vi "Repeatability_test.vi"(10 "PEU":refnum<class "PEU.lvclass">, 11 "E5071C":refnum<class "E5071C.lvclass">) -> ()   [LabVIEW 2020]
uses:
  Driver/E5071C/E5071C/E5071C.lvclass
  Driver/PEU/PEU/PEU.lvclass
  <vilib>/Math Plots/3D Math Plots/3D Scatter/3D Scatter XCtrl/3D Scatter.xctl
  <vilib>/Utility/NIReport.llb/Report Type.ctl
  Driver/E5071C/E5071C/E5071C.lvclass/E5071C.ctl
  <vilib>/addons/_office/excel.llb/Excel Get Data ([str]).vi
  <vilib>/Math Plots/3D Math Plots/3D Scatter/3D Scatter Datatype/Public/Plot Helper (Matrix).vi
  <vilib>/Utility/NIReport.llb/NI_report.lvclass
  <vilib>/Utility/NIReport.llb/NI_ReportGenerationCore.lvlib
  <vilib>/Utility/NIReport.llb/Excel/NI_Excel.lvclass
  <vilib>/addons/_office/NI_ReportGenerationToolkit.lvlib
  <instrlib>/Agilent ENA Series/Agilent ENA Series.lvlib
  <vilib>/Math Plots/3D Math Plots/3D Scatter/3D Scatter Datatype/3D Scatter Datatype.lvclass
panel:
  in  "循环次数":i32=1 min=1
  in  "引脚":string(combo)="SPDT"
  in  "Load":bool
  in  "Test":bool
  in  "Save":bool
  in  "负载选择":enum32{"Item 0", "Item 1"}(radio)
  in  "DUT ID:":string
  in  "DUT\n开关类型":string(combo)="SPDT"
  in  "Panel Show":bool
  in  "Tab Control":T1(tab)
  out "VSWR Graph":cluster{"频率":dbl[], dbl[]}[](graph)
  out "IL Graph":cluster{"Freqs":dbl[], "temp_value":dbl[]}[](graph)
  out "ISL Graph":cluster{"Freqs":dbl[], "temp_value":dbl[]}[](graph)
  out "VSWR(3D)":refnum<class "3D Plot Datatype.lvclass">[](xcontrol)
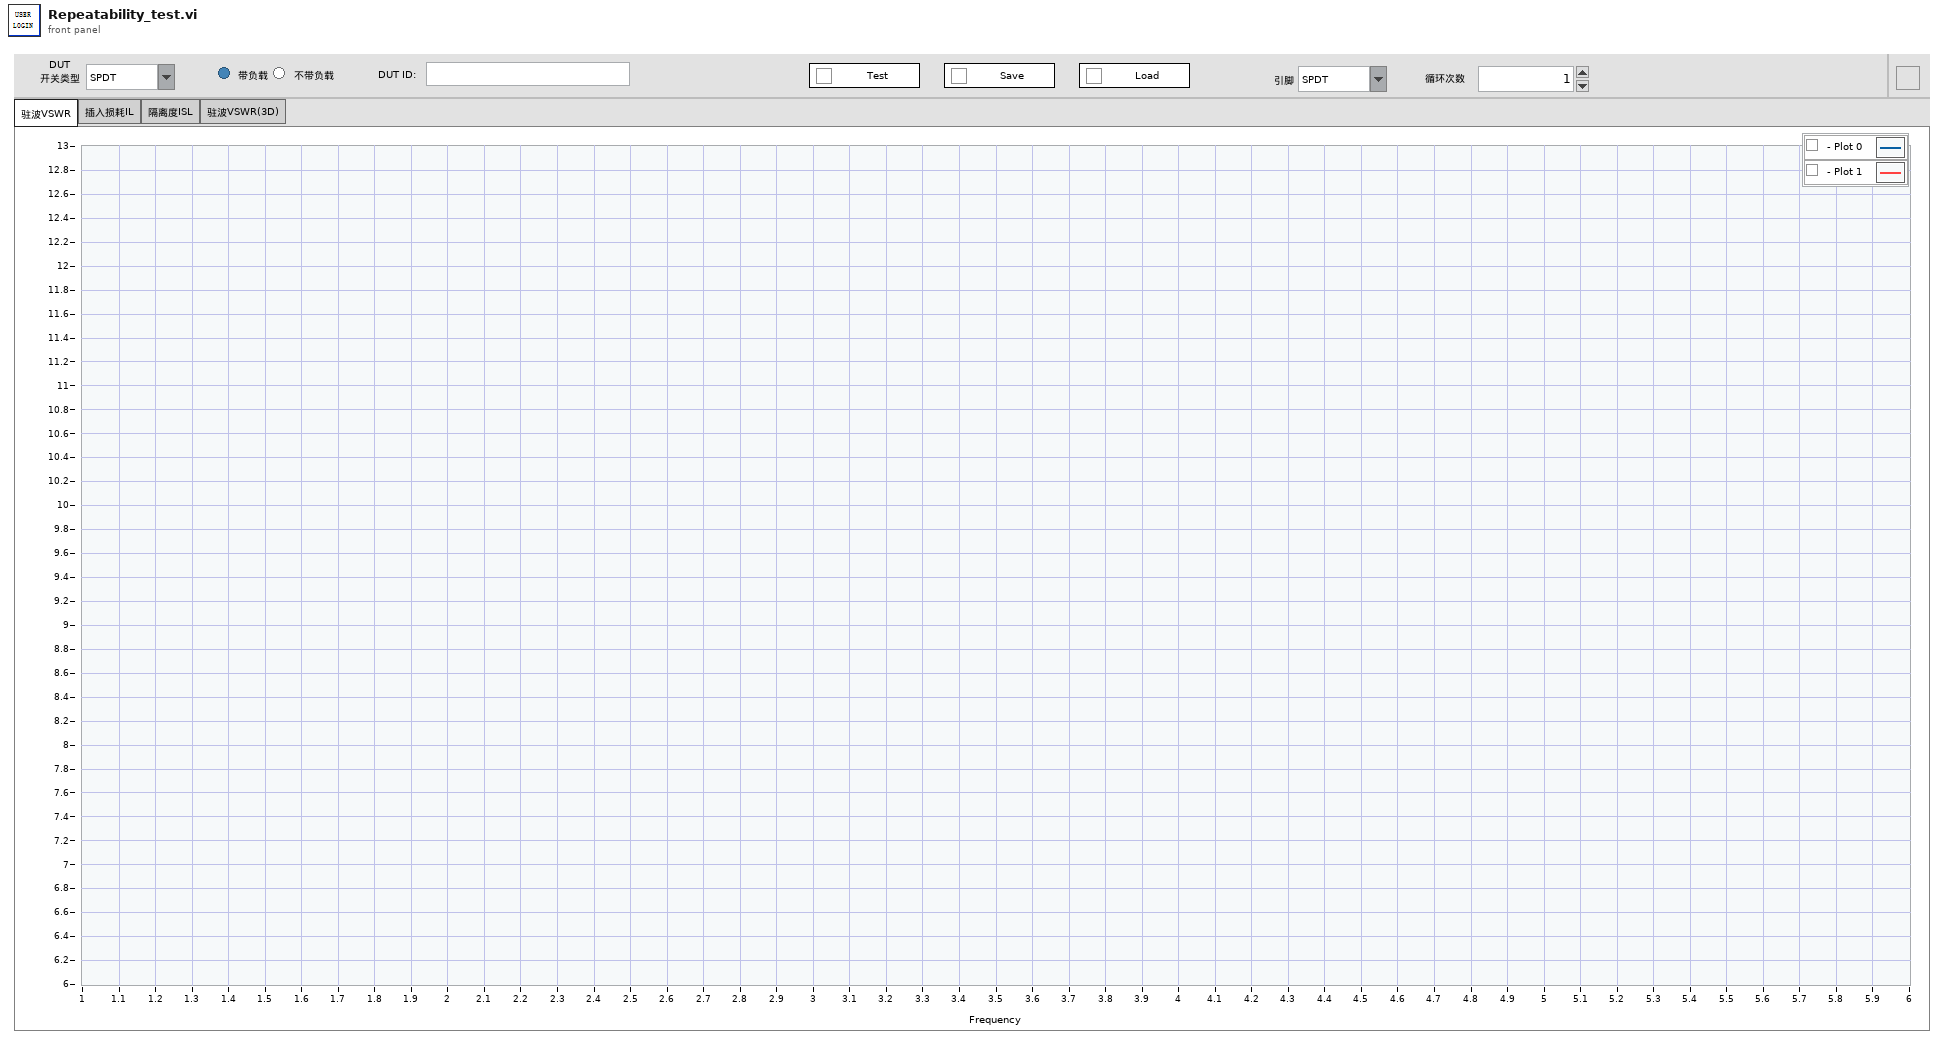
[diagram p1: front panel]
types:
  T1 = enum32{"驻波VSWR", "插入损耗IL", "隔离度ISL", "驻波VSWR(3D)"}
  T2 = enum32{"Invalid", "Standard", "Closed", "Hidden", "Minimized", "Maximized"}
  T3 = cluster{"校准文件":string[], "控制箱通道":string[], "DUT导通引脚":string[], "S名称":string[], "配置S":string[], "Plot_Name":string[]}
  T4 = typedef "NI_ReportGenerationCore.lvlib/Report Type.ctl" = enum16{"HTML", "Word", "Excel"}
  T5 = enum16{"maximized", "minimized", "normal", "no change"}
  T6 = cluster{"E5071C":refnum<class "E5071C.lvclass">, "PEU":refnum<class "PEU.lvclass">, "Index":i32, "Limit_Table":cluster{"Limit_IL":string[][], "Limit_VSWR":string[][], "Limit_ISL":string[][]}, "VSWR Graph":cluster{"频率":dbl[], dbl[]}[], "temp_value":dbl[], "Freqs":dbl[], "Count":i32, "测试逻辑":cluster{"校准文件":string[], "控制箱通道":string[], "DUT导通引脚":string[], "S名称":string[], "配置S":string[], "Plot_Name":string[]}, "VSWR_State":bool, "IL_State":bool, "ISL_State":bool, "循环次数":i32}
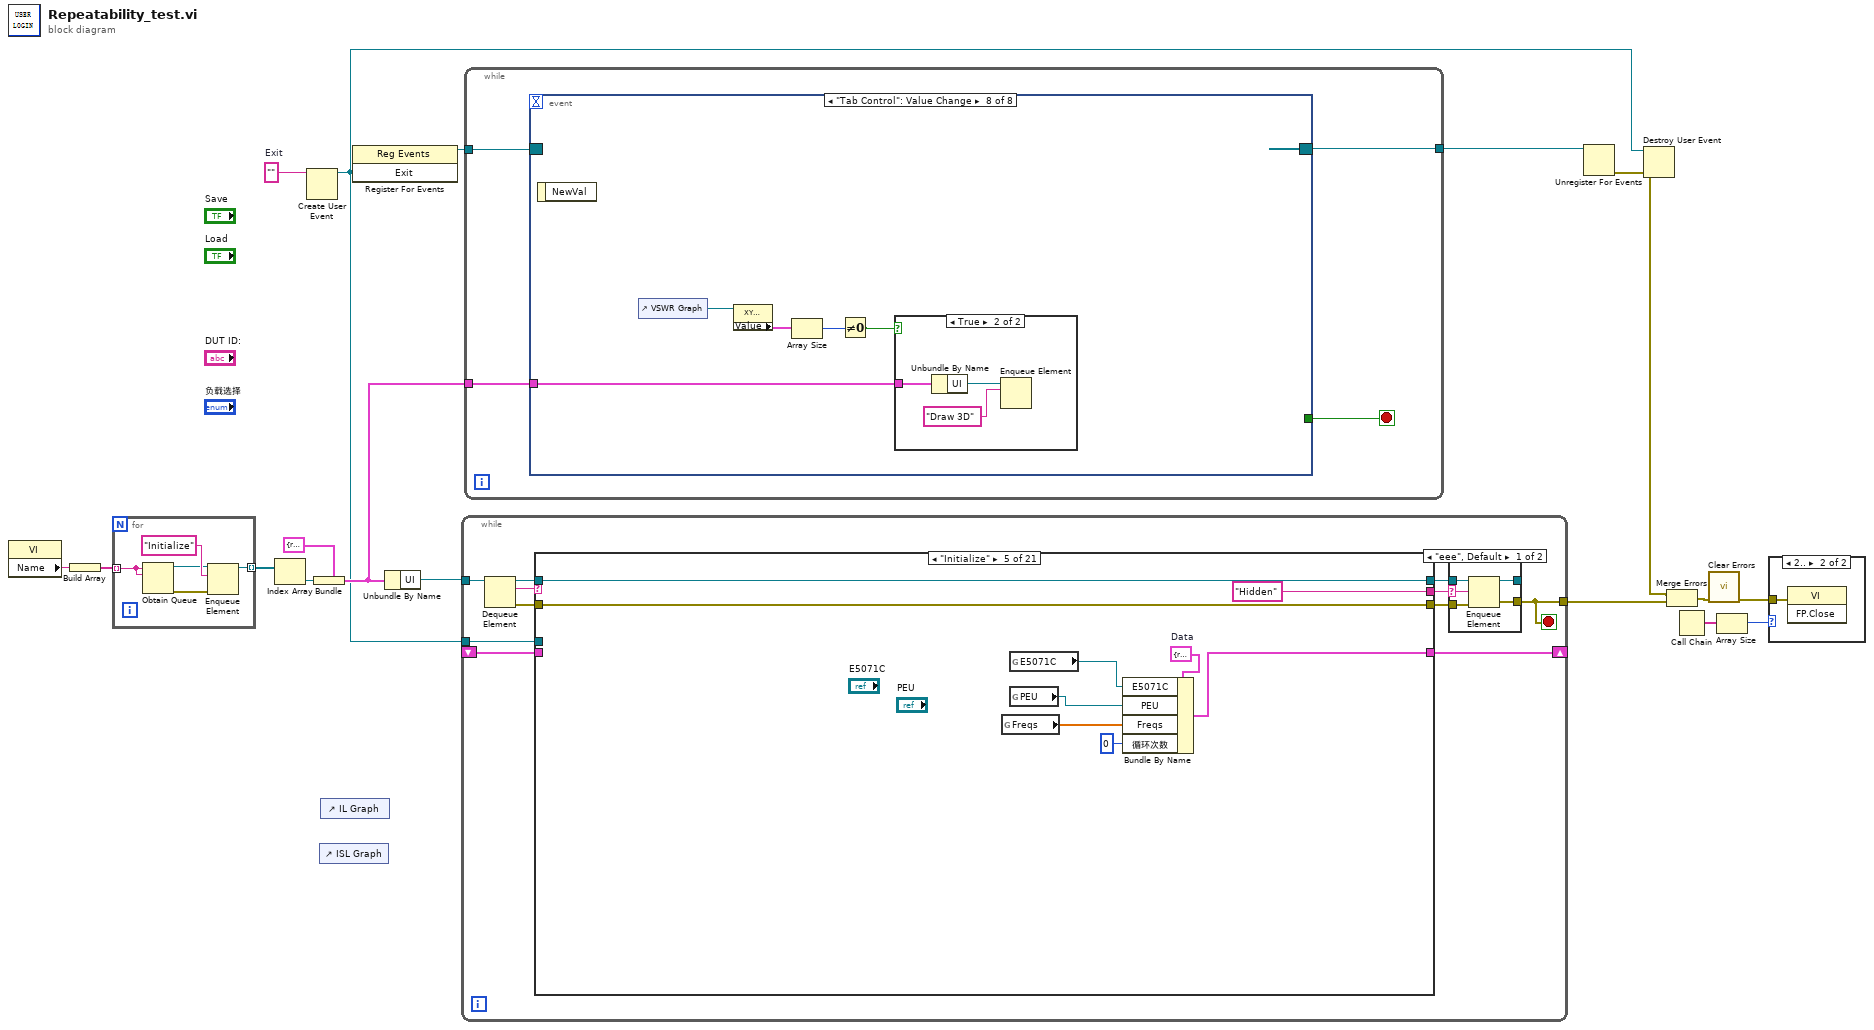
[diagram p0: block diagram]
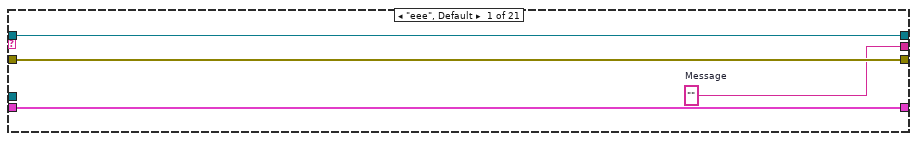
[diagram p4: hidden frame]
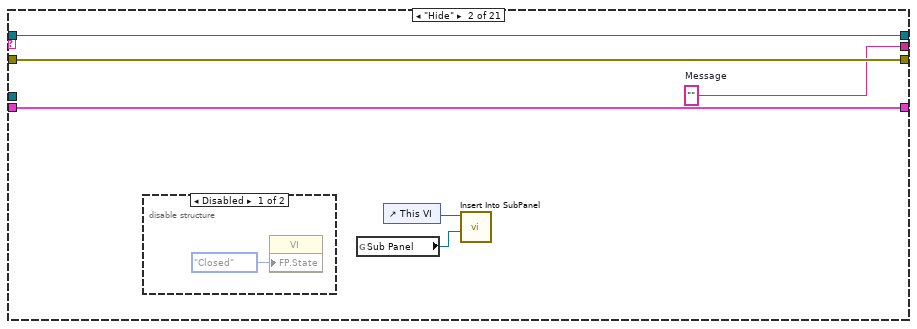
[diagram p5: hidden frame]
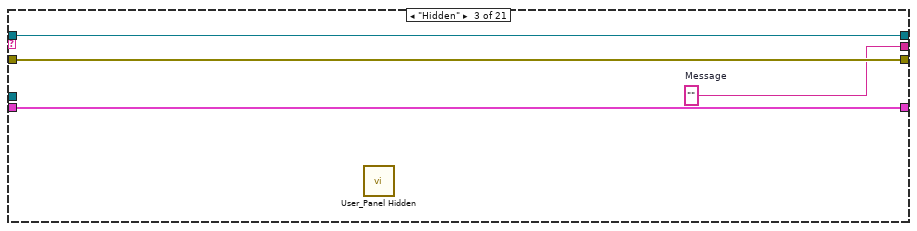
[diagram p7: hidden frame]
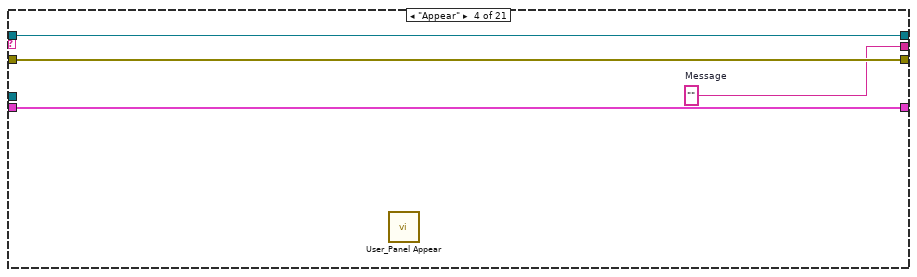
[diagram p8: hidden frame]
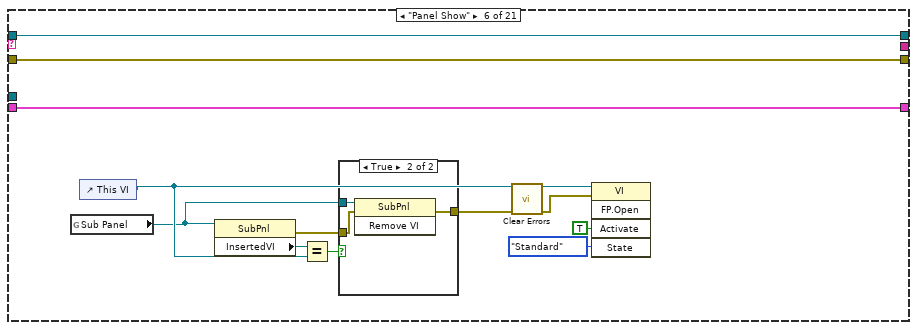
[diagram p9: hidden frame]
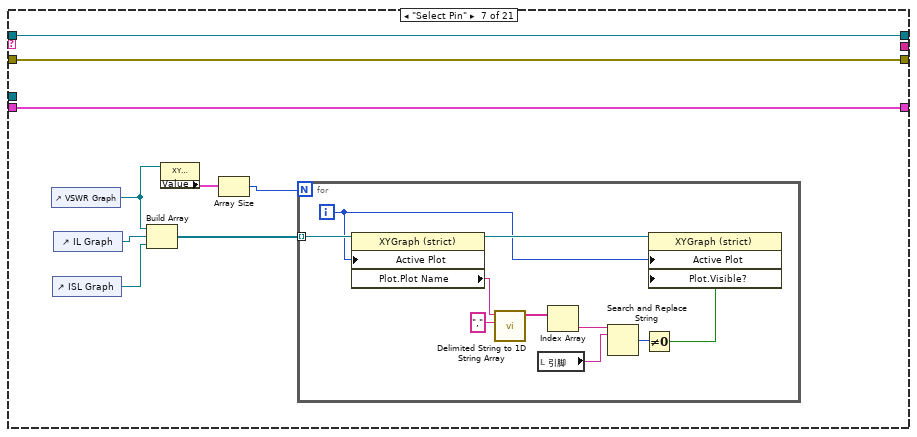
[diagram p11: hidden frame]
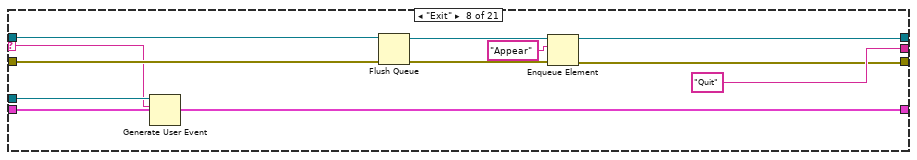
[diagram p12: hidden frame]
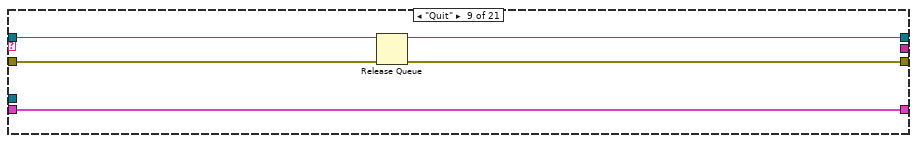
[diagram p13: hidden frame]
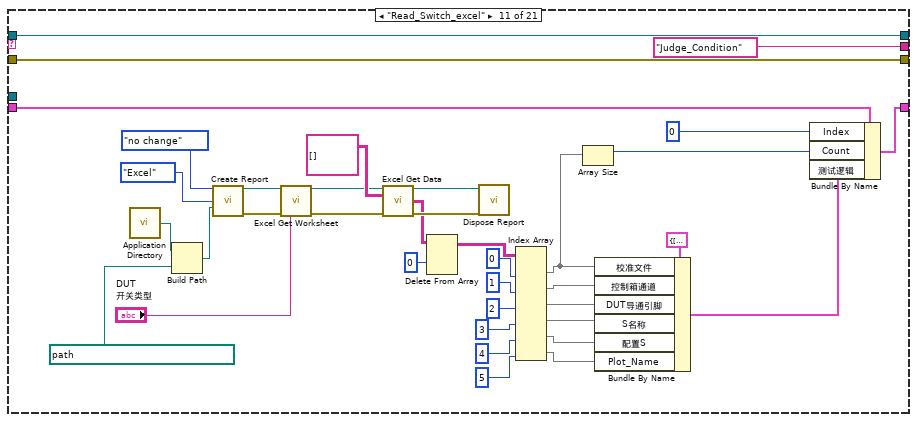
[diagram p15: hidden frame]
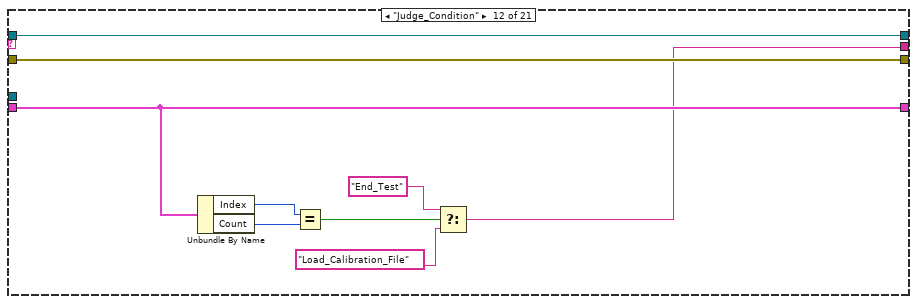
[diagram p16: hidden frame]
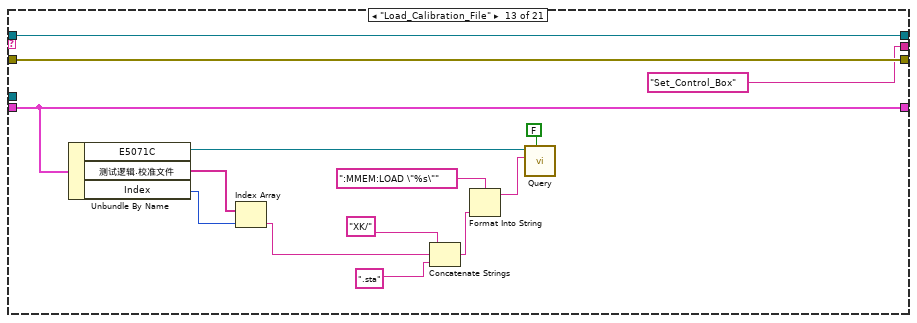
[diagram p17: hidden frame]
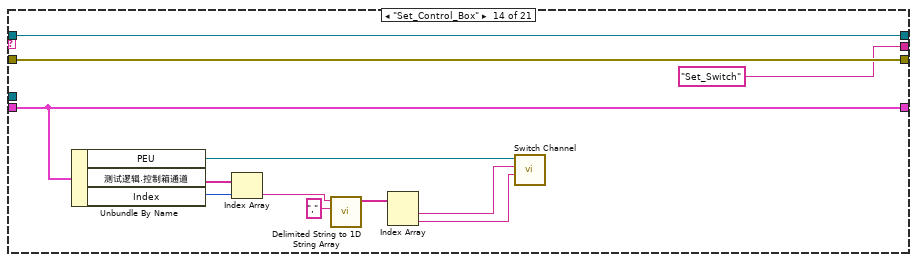
[diagram p18: hidden frame]
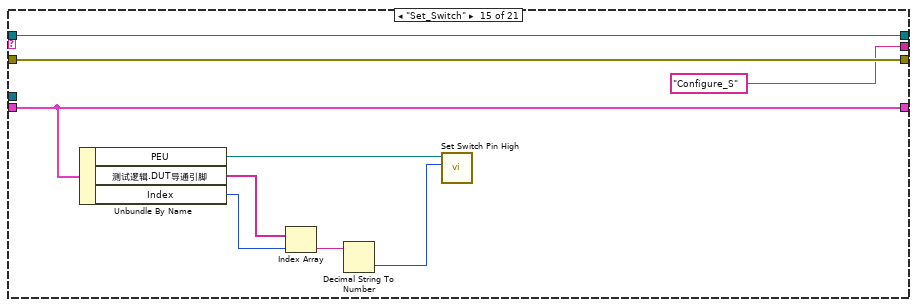
[diagram p19: hidden frame]
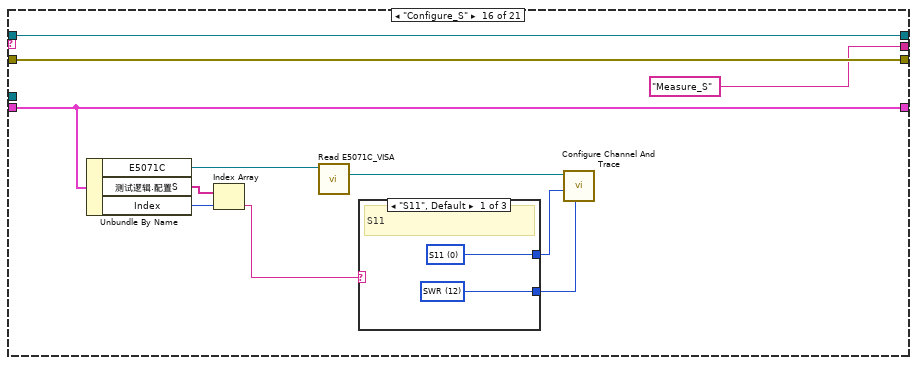
[diagram p20: hidden frame]
diagram:
  w7 = ""  # Exit
  n1 = property class="VI"() -> ("Name"=w17:string)  [unwired: 2 in, 2 out]
  n2 = Build Array(w17) -> (w18:string[])
  n3 = for {
    tunnel: w18 -> [w19] mode=indexing
    tunnel: [w20] -> w12 mode=indexing
    n4 = Obtain Queue(name (unnamed)=w19, element data type=w19) -> (queue out=w22:refnum<queue>, error out=w21:errorcluster)  [unwired: 3 in, 1 out]
    n5 = Enqueue Element(queue=w22, element="Initialize" ("元素"), error in (no error)=w21) -> (queue out=w20:refnum<queue>)  [unwired: 1 in, 2 out]
  }
  n6 = Index Array(array=w12) -> (element=w15:refnum<queue>)  [unwired: 1 in]
  n7 = Create User Event(user event datatype=w7) -> (user event=w11:refnum<user-event>)  [unwired: 1 in, 1 out]
  n8 = Bundle(cluster=cluster{"UI":refnum<queue>} {"UI"=refnum}, "UI"=w15) -> (w16:cluster{"UI":refnum<queue>})
  n9 = control-ref of="ISL Graph"() -> ()  [unwired: 1 out]
  n10 = control-ref of="IL Graph"() -> ()  [unwired: 1 out]
  n11 = register-events(w11) -> (reference out=w8:refnum<event-registration>)  [unwired: 2 in, 1 out]
  n12 = Unbundle By Name(w16) -> ("UI"=w13:refnum<queue>)
  n13 = while {
    tunnel: w13 -> [w34]
    tunnel: [w24] -> w1
    shift-right: [w28] -> _
    shift-left: _ -> [w27]
    tunnel: w11 -> [w26]
    stop <- w24 stop-if-true
    n14 = Dequeue Element(queue=w34) -> (queue out=w33:refnum<queue>, element=w25:string, error out=w30:errorcluster)  [unwired: 2 in, 1 out]
    n15 = case shown="\"Initialize\"" w25 {
      selector: w25 -> [_ _ _ _ _ _ _ w109 _ _ _ _ _ _ _ _ _ _ _ _ _]
      tunnel: w33 -> [w45 w51 w56 w60 w69 w81 w93 w112 w118 w121 w158 w167 w181 w193 w202 w213 w228 w255 w281 w288 w295]
      tunnel: [w45 w51 w56 w60 w69 w81 w93 w104 w118 w121 w158 w167 w181 w193 w202 w213 w228 w255 w281 w288 w295] -> w32
      tunnel: [w44 w50 w55 w59 w68 w80 w92 w105 w115 w120 w157 w166 w180 w192 w201 w212 w227 w254 w280 w287 w294] -> w31
      tunnel: w30 -> [w44 w50 w55 w59 w68 w80 w92 w111 w117 w120 w157 w166 w180 w192 w201 w212 w227 w254 w280 w287 w294]
      tunnel: [w43 w49 w54 w58 "Hidden" ("Message") _ _ "Quit" ("Message") _ _ "Judge_Condition" ("Message") w159 "Set_Control_Box" ("Message") "Set_Switch" ("Message") "Configure_S" ("Message") "Measure_S" ("Message") "Refresh_Graph" ("Message") "Judge_Condition" ("Message") w273 _ _] -> w29
      tunnel: [w42 w48 w53 w57 w67 w79 w91 w114 w116 w119 w130 w160 w169 w183 w195 w204 w221 w248 w278 w286 w290] -> w28
      tunnel: w27 -> [w42 w48 w53 w57 _ w79 w91 w114 w116 w119 w131 w160 w169 w183 w195 w204 w222 w248 w277 w286 w290]
      tunnel: w26 -> [_ _ _ _ _ _ _ w110 _ _ _ _ _ _ _ _ _ _ _ _ _]
      frame "eee", Default {
        w43 = ""  # Message
      }
      frame "Hide" {
        w49 = ""  # Message
        n16 = disable-structure shown="Disabled" {
          frame Disabled {
            n17 = property class="VI"("FP.State"=T2."Closed" ("前面板窗口:状态")) -> ()  [unwired: 2 in, 2 out]
          }
          frame Enabled {
          }
        }
        n18 = global read "Global.vi" "Sub Panel"() -> (w46:refnum<vi>)
        n19 = control-ref of="This VI"() -> (w47:refnum<vi>)
        n20 = call "Insert Into SubPanel.vi"("SubPanel Ref"=w46, "VI Ref In"=w47) -> ()  [unwired: 9 in, 1 out]
      }
      frame "Hidden" {
        w54 = ""  # Message
        n21 = call "User_Panel Hidden.vi"() -> ()  [unwired: 11 in, 1 out]
      }
      frame "Appear" {
        w58 = ""  # Message
        n22 = call "User_Panel Appear.vi"() -> ()  [unwired: 11 in, 1 out]
      }
      frame "Initialize" {
        w65 = T6 {"E5071C"=refnum, "PEU"=refnum, "Index"=0, "Limit_Table"={"Limit_IL"=[], "Limit_VSWR"=[], "Limit_ISL"=[]}, "VSWR Graph"=[], "temp_value"=[], "Freqs"=[], "Count"=0, "测试逻辑"={"校准文件"=[], "控制箱通道"=[], "DUT导通引脚"=[], "S名称"=[], "配置S"=[], "Plot_Name"=[]}, "VSWR_State"=FALSE, "IL_State"=FALSE, "ISL_State"=FALSE, "循环次数"=1}  # Data
        n23 = global read "Global.vi" "Freqs"() -> (w64:dbl[])
        n24 = global read "Global.vi" "E5071C"() -> (w62:refnum<class "E5071C.lvclass">)
        n25 = global read "Global.vi" "PEU"() -> (w61:refnum<class "PEU.lvclass">)
        n26 = Bundle By Name(cluster=w65, "E5071C"=w62, "PEU"=w61, "Freqs"=w64, "循环次数"=0) -> (w67:T6)
      }
      frame "Panel Show" {
        n27 = global read "Global.vi" "Sub Panel"() -> (w70:refnum<vi>)
        n28 = control-ref of="This VI"() -> (w71:refnum<vi>)
        n29 = property class="SubPnl"(reference=w70) -> (error out=w78:errorcluster, "InsertedVI"=w76:refnum<vi>)  [unwired: 1 in, 1 out]
        n30 = Equal?(x=w76, y=w71) -> (x = y?=w77:bool)
        n31 = case shown="True" w77 {
          tunnel: [_ w84] -> w72
          tunnel: w70 -> [_ w83]
          tunnel: w78 -> [_ w82]
          frame False {
          }
          frame True {
            n32 = invoke class="SubPnl" method="Remove VI"(reference=w83, error in=w82) -> (error out=w84:errorcluster)  [unwired: 1 in, 2 out]
          }
        }
        n33 = call <vilib>:"Clear Errors.vi"("error in (no error)"=w72) -> ("error out"=w75:errorcluster)  [unwired: 5 in, 1 out]
        n34 = invoke class="VI" method="FP.Open"(reference=w71, error in=w75, "Activate"=TRUE ("激活？"), "State"=T2."Standard" ("状态")) -> ()  [unwired: 1 in, 5 out]
      }
      frame "Select Pin" {
        n35 = control-ref of="VSWR Graph"() -> (w87:refnum<vi>)
        n36 = control-ref of="ISL Graph"() -> (w89:refnum<vi>)
        n37 = control-ref of="IL Graph"() -> (w90:refnum<vi>)
        n38 = Build Array(w87, w90, w89) -> (w88:refnum<vi>[])
        n39 = property class="XYGraph (strict)"(reference=w87) -> ("Value"=w86:cluster{"频率":dbl[], dbl[]}[])  [unwired: 1 in, 2 out]
        n40 = Array Size(array=w86) -> (size(s)=w85:i32)
        n41 = for {
          N: w85 -> [_]
          tunnel: w88 -> [w103] mode=indexing
          i -> [w101]
          n42 = property class="XYGraph (strict)"(reference=w103, "Active Plot"=w101) -> (reference out=w102:refnum<vi>, "Plot.Plot Name"=w100:string)  [unwired: 1 in, 1 out]
          n43 = call <vilib>:"Delimited String to 1D String Array.vi"("delimiter"=",", "delimited string"=w100) -> ("string array"=w98:string[])  [unwired: 9 in]
          n44 = local read "引脚"() -> (w96:string)
          n45 = Index Array(array=w98) -> (element=w97:string)  [unwired: 1 in]
          n46 = Search and Replace String(input string=w97, search string=w96) -> (number of replacements=w95:i32)  [unwired: 6 in, 3 out]
          n47 = Not Equal To 0?(x=w95) -> (x != 0?=w94:bool)
          n48 = property class="XYGraph (strict)"(reference=w102, "Active Plot"=w101, "Plot.Visible?"=w94) -> ()  [unwired: 1 in, 2 out]
        }
      }
      frame "Exit" {
        n49 = Generate User Event(user event=w110, event data cluster=w109) -> ()  [unwired: 2 in, 2 out]
        n50 = Flush Queue(queue=w112, error in (no error)=w111) -> (queue out=w107:refnum<queue>, error out=w106:errorcluster)  [unwired: 1 out]
        n51 = Enqueue Element(queue=w107, element="Appear" ("元素"), error in (no error)=w106) -> (queue out=w104:refnum<queue>, error out=w105:errorcluster)  [unwired: 1 in, 1 out]
      }
      frame "Quit" {
        n52 = Release Queue(queue=w118, error in (no error)=w117) -> (error out=w115:errorcluster)  [unwired: 1 in, 2 out]
      }
      frame "-------------Measurement-------------" {
      }
      frame "Read_Switch_excel" {
        n53 = call <vilib>:"Application Directory.vi"() -> ("Application Directory"=w132:path)
        n54 = Build Path(base path=w132, name or relative path=path "Config/开关映射表(重复性).xlsx") -> (appended path=w134:path)
        n55 = call <vilib>:"Create Report.vi"("window state (normal)"=T5."no change", "report type"=Report_Type."Excel", "template (empty)"=w134) -> ("report out"=w137:refnum<class "NI_report.lvclass">, "error out"=w138:errorcluster)  [unwired: 11 in]
        n56 = call <vilib>:"Excel Get Worksheet.vi"("report in"=w137, "error in (no error)"=w138, "name (\"\")"="DUT\n开关类型") -> ("report out"=w139:refnum<class "NI_report.lvclass">, "error out"=w140:errorcluster)  [unwired: 11 in]
        n57 = call-poly <vilib>:"Excel Get Data.vi"("report in"=w139, "data type"=string[][] [], "error in (no error)"=w140) -> ("report out"=w154:refnum<class "NI_report.lvclass">, "data"=w150:string[][], "error out"=w155:errorcluster)  [unwired: 10 in]
        n58 = Delete From Array(array=w150, index (row)=0) -> (array with subset deleted=w144:string[][])  [unwired: 2 in, 1 out]
        n59 = call-dynamic "Dispose Report.vi"("report in"=w154, "error in (no error)"=w155) -> ()  [unwired: 13 in, 1 out]
        n60 = Index Array(array=w144, index (col) #1=0 ("disabled index (col)"), index (col) #2=1 ("disabled index (col)"), index (col) #3=2 ("disabled index (col)"), index (col) #4=3 ("disabled index (col)"), index (col) #5=4 ("disabled index (col)"), index (col) #6=5 ("disabled index (col)")) -> (element #1=w151:string[], element #2=w148:string[], element #3=w149:string[], element #4=w124:string[], element #5=w123:string[], element #6=w122:string[])  [unwired: 6 in]
        n61 = Array Size(array=w151) -> (size(s)=w152:i32)
        n62 = Bundle By Name(cluster=T3 {"校准文件"=[], "控制箱通道"=[], "DUT导通引脚"=[], "S名称"=[], "配置S"=[], "Plot_Name"=[]}, "校准文件"=w151, "控制箱通道"=w148, "DUT导通引脚"=w149, "S名称"=w124, "配置S"=w123, "Plot_Name"=w122) -> (w153:T3)
        n63 = Bundle By Name(cluster=w131, "Index"=0, "Count"=w152, "测试逻辑"=w153) -> (w130:T6)
      }
      frame "Judge_Condition" {
        n64 = Unbundle By Name(w160) -> ("Index"=w161:i32, "Count"=w162:i32)
        n65 = Equal?(x=w161, y=w162) -> (x = y?=w163:bool)
        n66 = Select(t="End_Test", s=w163, f="Load_Calibration_File" ("Message")) -> (s? t:f=w159:string)
      }
      frame "Load_Calibration_File" {
        n67 = Unbundle By Name(w169) -> ("E5071C"=w170:refnum<class "E5071C.lvclass">, "测试逻辑.校准文件"=w176:string[], "Index"=w177:i32)
        n68 = Index Array(array=w176, index=w177) -> (element=w179:string)
        n69 = Concatenate Strings("XK/", w179, ".sta") -> (w173:string)
        n70 = Format Into String(format string=":MMEM:LOAD \"%s\"" ("Command"), w173) -> (resulting string=w175:string)  [unwired: 2 in, 1 out]
        n71 = call "Query.vi"("Return"=FALSE, "Command"=w175, "E5071C in"=w170) -> ()  [unwired: 6 in, 3 out]
      }
      frame "Set_Control_Box" {
        n72 = Unbundle By Name(w183) -> ("PEU"=w184:refnum<class "PEU.lvclass">, "测试逻辑.控制箱通道"=w185:string[], "Index"=w186:i32)
        n73 = Index Array(array=w185, index=w186) -> (element=w187:string)
        n74 = call <vilib>:"Delimited String to 1D String Array.vi"("delimiter"=",", "delimited string"=w187) -> ("string array"=w189:string[])  [unwired: 9 in]
        n75 = Index Array(array=w189) -> (element #1=w190:string, element #2=w191:string)  [unwired: 2 in]
        n76 = call "Switch Channel.vi"("CH2"=w191, "CH1"=w190, "PEU in"=w184) -> ()  [unwired: 7 in, 2 out]
      }
      frame "Set_Switch" {
        n77 = Unbundle By Name(w195) -> ("PEU"=w198:refnum<class "PEU.lvclass">, "测试逻辑.DUT导通引脚"=w196:string[], "Index"=w197:i32)
        n78 = Index Array(array=w196, index=w197) -> (element=w199:string)
        n79 = Decimal String To Number(string=w199) -> (number=w200:i32)  [unwired: 2 in, 1 out]
        n80 = call "Set Switch Pin High.vi"("Pin"=w200, "PEU in"=w198) -> ()  [unwired: 8 in, 2 out]
      }
      frame "Configure_S" {
        n81 = Unbundle By Name(w204) -> ("E5071C"=w205:refnum<class "E5071C.lvclass">, "测试逻辑.配置S"=w209:string[], "Index"=w210:i32)
        n82 = Index Array(array=w209, index=w210) -> (element=w211:string)
        n83 = call "Read E5071C_VISA.vi"("E5071C in"=w205) -> ("E5071C_VISA"=w206:refnum<visa-resource-name>)  [unwired: 8 in, 2 out]
        n84 = case shown="\"S11\", Default" w211 {
          tunnel: [w215 w216 w219] -> w207
          tunnel: [w214 w217 w218] -> w208
          frame "S11", Default {
            w215 = u16 12 items=["Logarithmic Magnitude", "Phase", "Group Delay", "Smith Chart  Linear (Lin/Phase)", "Smith Chart  Logarithmic (Log/Phase)", "Smith Chart  Complex (Real/Imag)", "Smith Chart  Impedance (R+jX)", "Smith Chart  Admittance (G+jB)", "Polar Format (Linear)", "Polar Format (Logarithmic)", "Polar Format (Re/Im)", "Linear Magnitude", "SWR", "Real", "Imaginary", "Epanded Phase", "Positive Phase"] ("Data Format (0: Logarithmic Magnitude)")
            w214 = u16 0 items=["S11", "S21", "S31", "S41", "S12", "S22", "S32", "S42", "S13", "S23", "S33", "S43", "S14", "S24", "S34", "S44", "A", "B", "C", "D", "R1", "R2", "R3", "R4", "AUX1", "AUX2", "TR", "T", "R"] ("Measurement Parameters (0: S11)")
            # "S11"
          }
          frame "S21" {
            w216 = u16 0 items=["Logarithmic Magnitude", "Phase", "Group Delay", "Smith Chart  Linear (Lin/Phase)", "Smith Chart  Logarithmic (Log/Phase)", "Smith Chart  Complex (Real/Imag)", "Smith Chart  Impedance (R+jX)", "Smith Chart  Admittance (G+jB)", "Polar Format (Linear)", "Polar Format (Logarithmic)", "Polar Format (Re/Im)", "Linear Magnitude", "SWR", "Real", "Imaginary", "Epanded Phase", "Positive Phase"] ("Data Format (0: Logarithmic Magnitude)")
            w217 = u16 1 items=["S11", "S21", "S31", "S41", "S12", "S22", "S32", "S42", "S13", "S23", "S33", "S43", "S14", "S24", "S34", "S44", "A", "B", "C", "D", "R1", "R2", "R3", "R4", "AUX1", "AUX2", "TR", "T", "R"] ("Measurement Parameters (0: S11)")
            # "S21(IL)"
          }
          frame "S22" {
            w219 = u16 12 items=["Logarithmic Magnitude", "Phase", "Group Delay", "Smith Chart  Linear (Lin/Phase)", "Smith Chart  Logarithmic (Log/Phase)", "Smith Chart  Complex (Real/Imag)", "Smith Chart  Impedance (R+jX)", "Smith Chart  Admittance (G+jB)", "Polar Format (Linear)", "Polar Format (Logarithmic)", "Polar Format (Re/Im)", "Linear Magnitude", "SWR", "Real", "Imaginary", "Epanded Phase", "Positive Phase"] ("Data Format (0: Logarithmic Magnitude)")
            w218 = u16 5 items=["S11", "S21", "S31", "S41", "S12", "S22", "S32", "S42", "S13", "S23", "S33", "S43", "S14", "S24", "S34", "S44", "A", "B", "C", "D", "R1", "R2", "R3", "R4", "AUX1", "AUX2", "TR", "T", "R"] ("Measurement Parameters (0: S11)")
            # "S22"
          }
        }
        n85 = call <instrlib>:"Configure Channel And Trace.vi"("Data Format (0: Logarithmic Magnitude)"=w207, "Measurement Parameters (0: S11)"=w208, "VISA resource name"=w206) -> ()  [unwired: 7 in, 2 out]
      }
      frame "Measure_S" {
        n86 = Unbundle By Name(w222) -> ("E5071C"=w223:refnum<class "E5071C.lvclass">, "Freqs"=w225:dbl[])
        n87 = call "Read E5071C_VISA.vi"("E5071C in"=w223) -> ("E5071C_VISA"=w224:refnum<visa-resource-name>)  [unwired: 8 in, 2 out]
        n88 = for {
          tunnel: w224 -> [w231]
          tunnel: w225 -> [w230] mode=indexing
          tunnel: [w229] -> w226 mode=indexing
          n89 = call <instrlib>:"Set Marker Position.vi"("X Value (0.0)"=w230, "VISA resource name"=w231) -> ("error out"=w232:errorcluster, "VISA resource name out"=w233:refnum<visa-resource-name>)  [unwired: 8 in]
          n90 = call <instrlib>:"Marker Data.vi"("error in (no error)"=w232, "VISA resource name"=w233) -> ("Y Real Value"=w229:dbl)  [unwired: 5 in, 4 out]
        }
        n91 = Bundle By Name(cluster=w222, "temp_value"=w226) -> (w221:T6)
      }
      frame "Refresh_Graph" {
        n92 = Unbundle By Name(w248) -> ("测试逻辑.S名称"=w249:string[], "Index"=w236:i32, "Freqs"=w251:dbl[], "temp_value"=w252:dbl[], "测试逻辑.Plot_Name"=w242:string[], "测试逻辑.DUT导通引脚"=w237:string[])
        n93 = Index Array(array=w249, index=w236) -> (element=w250:string)
        n94 = Bundle("Freqs"=w251, "temp_value"=w252) -> (w253:cluster{"Freqs":dbl[], "temp_value":dbl[]})  [unwired: 1 in]
        n95 = Index Array(array=w237, index=w236) -> (element=w235:string)
        n96 = Index Array(array=w242, index=w236) -> (element=w241:string)
        n97 = case shown="\"插损\"" w250 {
          tunnel: w253 -> [w259 w264 w269]
          tunnel: [w256 w261 w266] -> w240
          frame "驻波", Default {
            # "S11、S22"
            n98 = control-ref of="VSWR Graph"() -> (w258:refnum<vi>)
            n99 = property class="XYGraph (strict)"(reference=w258) -> (reference out=w256:refnum<vi>, "Value"=w260:cluster{"频率":dbl[], dbl[]}[])  [unwired: 1 in, 1 out]
            n100 = Build Array (concatenate)(w260, w259) -> (→"VSWR Graph":cluster{"Freqs":dbl[], "temp_value":dbl[]}[])
          }
          frame "插损" {
            # "S21(IL)"
            n101 = control-ref of="IL Graph"() -> (w262:refnum<vi>)
            n102 = property class="XYGraph (strict)"(reference=w262) -> (reference out=w261:refnum<vi>, "Value"=w265:cluster{"Freqs":dbl[], "temp_value":dbl[]}[])  [unwired: 1 in, 1 out]
            n103 = Build Array (concatenate)(w265, w264) -> (→"IL Graph":cluster{"Freqs":dbl[], "temp_value":dbl[]}[])
          }
          frame "隔离" {
            # "S21(ISO)"
            n104 = control-ref of="ISL Graph"() -> (w267:refnum<vi>)
            n105 = property class="XYGraph (strict)"(reference=w267) -> (reference out=w266:refnum<vi>, "Value"=w270:cluster{"Freqs":dbl[], "temp_value":dbl[]}[])  [unwired: 1 in, 1 out]
            n106 = Build Array (concatenate)(w270, w269) -> (→"ISL Graph":cluster{"Freqs":dbl[], "temp_value":dbl[]}[])
          }
        }
        n107 = property class="XYGraph (strict)"(reference=w240) -> (reference out=w243:refnum<vi>, "LegNumRows"=w245:u32)  [unwired: 1 in, 1 out]
        n108 = Search and Replace String(input string="引脚", search string=w235) -> (number of replacements=w239:i32)  [unwired: 6 in, 3 out]
        n109 = Increment(x=w245) -> (x+1=w244:u32)
        n110 = Not Equal To 0?(x=w239) -> (x != 0?=w234:bool)
        n111 = property class="XYGraph (strict)"(reference=w243, "LegNumRows"=w244, "Active Plot"=w245, "Plot.Plot Name"=w241, "Plot.Line Width"=u8 2, "Plot.Visible?"=w234) -> ()  [unwired: 1 in, 2 out]
      }
      frame "End_Test" {
        n112 = Unbundle By Name(w277) -> ("循环次数"=w276:i32)
        n113 = Increment(x=w276) -> (x+1=w271:i32)
        n114 = Equal?(x=w271, y="循环次数") -> (x = y?=w274:bool)
        n115 = case shown="False" w274 {
          tunnel: ["Judge_Condition" ""] -> w273
          tunnel: [w282 0 ("Index")] -> w272
          tunnel: w271 -> [w282 _]
          frame False {
          }
          frame True {
          }
        }
        n116 = Bundle By Name(cluster=w277, "Index"=0, "循环次数"=w272) -> (w278:T6)
      }
      frame "-----------------3D-----------------" {
      }
      frame "Draw 3D" {
        n117 = local read "循环次数"() -> (w292:i32)
        n118 = Unbundle By Name(w290) -> ("Freqs"=w289:dbl[])
        n119 = for {
          N: w292 -> [_]
          tunnel: [w296] -> w291 mode=indexing
          i -> [w297]
          n120 = Increment(x=w297) -> (x+1=w296:i32)
        }
        n121 = case shown="\"驻波VSWR(3D)\"" "Tab Control" {
          tunnel: w291 -> [_ w304]
          tunnel: w289 -> [_ w303]
          frame "驻波VSWR", Default {
          }
          frame "驻波VSWR(3D)" {
            n122 = control-ref of="VSWR Graph"() -> (w300:refnum<vi>)
            n123 = property class="XYGraph (strict)"(reference=w300) -> (reference out=w302:refnum<vi>, "Value"=w301:cluster{"频率":dbl[], dbl[]}[])  [unwired: 1 in, 1 out]
            n124 = Array Size(array=w301) -> (size(s)=w299:i32)
            n125 = for {
              N: w299 -> [_]
              tunnel: w302 -> [w316]
              tunnel: w301 -> [w307] mode=indexing
              tunnel: [w306] -> w298 mode=indexing if=w308
              i -> [w309]
              n126 = property class="XYGraph (strict)"(reference=w316, "Active Plot"=w309) -> ("Plot.Plot Name"=w315:string)  [unwired: 1 in, 2 out]
              n127 = call <vilib>:"Delimited String to 1D String Array.vi"("delimiter"=",", "delimited string"=w315) -> ("string array"=w313:string[])  [unwired: 9 in]
              n128 = local read "引脚"() -> (w311:string)
              n129 = Index Array(array=w313) -> (element=w312:string)  [unwired: 1 in]
              n130 = Search and Replace String(input string=w312, search string=w311) -> (number of replacements=w310:i32)  [unwired: 6 in, 3 out]
              n131 = Not Equal To 0?(x=w310) -> (x != 0?=w308:bool)
              n132 = Unbundle(w307) -> (w306:dbl[])  [unwired: 1 out]
            }
            n133 = call-poly <vilib>:"Plot Helper.vi"("z matrix"=w298, "y vector"=w303, "x vector"=w304) -> ("3D Plot lvclass Array out"=→"VSWR(3D)":refnum<class "3D Plot Datatype.lvclass">[])  [unwired: 3 in, 5 out]
          }
        }
      }
    }
    n134 = case shown="\"eee\", Default" w29 {
      selector: w29 -> [w35 _]
      tunnel: w32 -> [w39 w41]
      tunnel: w31 -> [w38 w40]
      tunnel: [w37 w40] -> w24
      tunnel: [w36 w41] -> _
      frame "eee", Default {
        n135 = Enqueue Element(queue=w39, element=w35, error in (no error)=w38) -> (queue out=w36:refnum<queue>, error out=w37:errorcluster)  [unwired: 1 in, 1 out]
      }
      frame "" {
      }
    }
  }
  n136 = while {
    tunnel: w8 -> [w319]
    tunnel: [w318] -> w10
    tunnel: w16 -> [w317]
    stop <- w320 stop-if-true
    n137 = event shown="[7] \"Tab Control\": Value Change" {
      selector: w319 -> [_ _ _ _ _ _ _ _]
      dyn-events: [_ _ _ _ _ _ _ _] -> w318
      timeout: _ -> [_ _ _ _ _ _ _ _]
      tunnel: [_ _ _ _ _ w335 _ _] -> w320
      tunnel: w317 -> [_ _ w327 w330 w331 _ w339 w347]
      event Timeout {
        n138 = event-data() -> ()  [unwired: 1 in, 1 out]
      }
      event Key Down {
        n139 = event-data() -> ("Char"=w322:i16, "PlatMods.Ctrl"=w321:bool)  [unwired: 1 in]
        n140 = case shown="True" w321 {
          tunnel: w322 -> [_ w323]
          frame False {
          }
          frame True {
            n141 = case shown="101" w323 {
              frame 0, Default {
              }
              frame 101 {
                n142 = property class="VI"("BDWin.Open"=TRUE ("程序框图窗口:打开")) -> ()  [unwired: 2 in, 2 out]
              }
            }
          }
        }
      }
      event "Panel Show": Value Change {
        n143 = event-data() -> ()  [unwired: 1 in, 1 out]
        n144 = Unbundle By Name(w327) -> ("UI"=w326:refnum<queue>)
        n145 = Enqueue Element(queue=w326, element="Panel Show" ("元素")) -> ()  [unwired: 2 in, 3 out]
      }
      event "Test": Value Change {
        n146 = event-data() -> ()  [unwired: 1 in, 1 out]
        n147 = Unbundle By Name(w330) -> ("UI"=w329:refnum<queue>)
        n148 = Enqueue Element(queue=w329, element="Test" ("元素")) -> ()  [unwired: 2 in, 3 out]
      }
      event "引脚": Value Change {
        n149 = event-data() -> ()  [unwired: 1 in, 1 out]
        n150 = Unbundle By Name(w331) -> ("UI"=w333:refnum<queue>)
        n151 = Enqueue Element(queue=w333, element="Select Pin" ("元素")) -> ()  [unwired: 2 in, 3 out]
      }
      event User Event {
        n152 = event-data() -> ("Exit"=w336:string)  [unwired: 1 in]
        n153 = Equal?(x=w336, y="Exit") -> (x = y?=w335:bool)
      }
      event Panel Close? {
        n154 = event-data() -> ()  [unwired: 1 in, 1 out]
        n155 = Cluster To Array(cluster=w339) -> (array=w338:refnum<queue>[])
        n156 = for {
          tunnel: w338 -> [w342] mode=indexing
          tunnel: "Hide" ("元素") -> [w341]
          n157 = Enqueue Element(queue=w342, element=w341) -> ()  [unwired: 2 in, 3 out]
        }
        n158 = event-data("Discard?"=TRUE ("放弃？")) -> ()  [unwired: 1 in, 1 out]
      }
      event "Tab Control": Value Change {
        n159 = event-data() -> ()  [unwired: 1 in, 1 out]
        n160 = control-ref of="VSWR Graph"() -> (w346:refnum<vi>)
        n161 = property class="XYGraph (strict)"(reference=w346) -> ("Value"=w345:cluster{"频率":dbl[], dbl[]}[])  [unwired: 1 in, 2 out]
        n162 = Array Size(array=w345) -> (size(s)=w344:i32)
        n163 = Not Equal To 0?(x=w344) -> (x != 0?=w343:bool)
        n164 = case shown="True" w343 {
          tunnel: w347 -> [_ w348]
          frame False {
          }
          frame True {
            n165 = Unbundle By Name(w348) -> ("UI"=w350:refnum<queue>)
            n166 = Enqueue Element(queue=w350, element="Draw 3D" ("元素")) -> ()  [unwired: 2 in, 3 out]
          }
        }
      }
    }
  }
  n167 = Unregister For Events(event registration refnum=w10) -> (error out=w9:errorcluster)  [unwired: 1 in]
  n168 = Destroy User Event(user event=w11, error in=w9) -> (error out=w2:errorcluster)
  n169 = Merge Errors(w2, w1) -> (w6:errorcluster)
  n170 = Call Chain() -> (call chain=w4:string[])
  n171 = call <vilib>:"Clear Errors.vi"("error in (no error)"=w6) -> ("error out"=w5:errorcluster)  [unwired: 5 in, 1 out]
  n172 = Array Size(array=w4) -> (size(s)=w3:i32)
  n173 = case shown="2.." w3 {
    tunnel: w5 -> [_ w351]
    frame 0, Default {
    }
    frame 2.. {
      n174 = invoke class="VI" method="FP.Close"(error in=w351) -> ()  [unwired: 2 in, 3 out]
    }
  }
